vi "BMU诊断标定.vi"(8 "CAN端口":u16(ring), 9 "设备索引号":u16(ring), 10 "CAN卡类型":u32(ring)=21) -> ()   [LabVIEW 2013] (continued)
                n1433 = Build Array(w1898, w1897, w1896, w1895, w1894, w1893) -> (w1899:bool[])
                n1434 = Build Array(w1907, w1906, w1905, w1904, w1903, w1902) -> (w1901:bool[])
                n1435 = And Array Elements(Boolean array=w1899) -> (logical AND=w1892:bool)
                n1436 = And Array Elements(Boolean array=w1901) -> (logical AND=w1900:bool)
                n1437 = Not(x=w1891) -> (.not. x?=w1915:bool)
              }
              frame "电池包信息1" {
                w1920 = 2
                w1928 = 2
                w1919 = 2
                w1917 = FALSE ("1 6")
                n1438 = Select(t=0, s=w1925, f=1) -> (s? t:f=w1918:i32)
                n1439 = property on="串联数" class="DigNum (严格)"("Disabled"=w1918) -> ()  [unwired: 2 in, 2 out]
                n1440 = property on="并联数" class="DigNum (严格)"("Disabled"=w1918) -> ()  [unwired: 2 in, 2 out]
                n1441 = property on="电池厂家" class="DigNum (严格)"("Disabled"=w1918) -> ()  [unwired: 2 in, 2 out]
                n1442 = property on="电池类型" class="DigNum (严格)"("Disabled"=w1918) -> ()  [unwired: 2 in, 2 out]
                n1443 = property on="额定能量" class="DigNum (严格)"("Disabled"=w1918) -> ()  [unwired: 2 in, 2 out]
                n1444 = property on="额定容量" class="DigNum (严格)"("Disabled"=w1918) -> ()  [unwired: 2 in, 2 out]
                n1445 = property on="实际容量" class="DigNum (严格)"("Disabled"=w1918) -> ()  [unwired: 2 in, 2 out]
                n1446 = property on="电池组信息" class="Clust (严格)"("Disabled"=w1918) -> ()  [unwired: 2 in, 2 out]
                n1447 = property on="生产日期" class="Str"("DisabledEnum"=w1918) -> ()  [unwired: 2 in, 2 out]
                n1448 = property on="车牌号" class="Str"("DisabledEnum"=w1919) -> ()  [unwired: 2 in, 2 out]
                n1449 = property on="产权标识" class="DigNum (严格)"("Disabled"=w1918) -> ()  [unwired: 2 in, 2 out]
                n1450 = property on="应用车型" class="DigNum (严格)"("Disabled"=w1918) -> ()  [unwired: 2 in, 2 out]
                n1451 = property on="额定总压" class="DigNum (严格)"("Disabled"=w1918) -> ()  [unwired: 2 in, 2 out]
                n1452 = property on="电池包序号" class="DigNum (严格)"("DisabledEnum"=w1918) -> ()  [unwired: 2 in, 2 out]
                n1453 = property on="电池包组号" class="DigNum (严格)"("DisabledEnum"=w1919) -> ()  [unwired: 2 in, 2 out]
                n1454 = property on="最大允许单体电压" class="DigNum (严格)"("Disabled"=w1928) -> ()  [unwired: 2 in, 2 out]
                n1455 = property on="最大允许总电压" class="DigNum (严格)"("Disabled"=w1928) -> ()  [unwired: 2 in, 2 out]
                n1456 = property on="最大允许温度" class="DigNum (严格)"("Disabled"=w1928) -> ()  [unwired: 2 in, 2 out]
                n1457 = property on="最小允许温度" class="DigNum (严格)"("Disabled"=w1928) -> ()  [unwired: 2 in, 2 out]
                n1458 = property on="最大允许充电电流" class="DigNum (严格)"("Disabled"=w1928) -> ()  [unwired: 2 in, 2 out]
                n1459 = property on="最小允许充电电流" class="DigNum (严格)"("Disabled"=w1928) -> ()  [unwired: 2 in, 2 out]
                n1460 = property on="最小允许单体电压" class="DigNum (严格)"("Disabled"=w1928) -> ()  [unwired: 2 in, 2 out]
                n1461 = property on="电流步长" class="DigNum (严格)"("Disabled"=w1928) -> ()  [unwired: 2 in, 2 out]
                n1462 = property on="SOC" class="DigNum (严格)"("Disabled"=w1928) -> ()  [unwired: 2 in, 2 out]
                n1463 = property on="充电总安时" class="DigNum (严格)"("Disabled"=w1928) -> ()  [unwired: 2 in, 2 out]
                n1464 = property on="放电总安时" class="DigNum (严格)"("Disabled"=w1928) -> ()  [unwired: 2 in, 2 out]
                n1465 = property on="放空次数" class="DigNum (严格)"("DisabledEnum"=w1920) -> ()  [unwired: 2 in, 2 out]
                n1466 = property on="充满次数" class="DigNum (严格)"("DisabledEnum"=w1920) -> ()  [unwired: 2 in, 2 out]
                n1467 = property on="充电次数" class="DigNum (严格)"("DisabledEnum"=w1920) -> ()  [unwired: 2 in, 2 out]
                n1468 = global read "功能码全局.vi" "24"() -> (w1923:bool[])
                n1469 = global read "功能码全局.vi" "23"() -> (w1924:bool[])
                n1470 = Index Array(array=w1923) -> (element #3=w1921:bool)  [unwired: 8 in, 7 out]
                n1471 = Index Array(array=w1924) -> (element #3=w1922:bool)  [unwired: 8 in, 7 out]
                n1472 = Not(x=w1917) -> (.not. x?=w1929:bool)
              }
              frame "电池包组号" {
                w1934 = 2
                w1933 = 2
                w1943 = 2
                w1935 = 2
                w1944 = 2
                w1931 = FALSE ("1 6")
                n1473 = property on="串联数" class="DigNum (严格)"("Disabled"=w1944) -> ()  [unwired: 2 in, 2 out]
                n1474 = property on="并联数" class="DigNum (严格)"("Disabled"=w1944) -> ()  [unwired: 2 in, 2 out]
                n1475 = property on="电池厂家" class="DigNum (严格)"("Disabled"=w1944) -> ()  [unwired: 2 in, 2 out]
                n1476 = property on="电池类型" class="DigNum (严格)"("Disabled"=w1944) -> ()  [unwired: 2 in, 2 out]
                n1477 = property on="额定能量" class="DigNum (严格)"("Disabled"=w1944) -> ()  [unwired: 2 in, 2 out]
                n1478 = property on="额定容量" class="DigNum (严格)"("Disabled"=w1944) -> ()  [unwired: 2 in, 2 out]
                n1479 = property on="实际容量" class="DigNum (严格)"("Disabled"=w1944) -> ()  [unwired: 2 in, 2 out]
                n1480 = Select(t=0, s=w1940, f=1) -> (s? t:f=w1932:i32)
                n1481 = property on="生产日期" class="Str"("DisabledEnum"=w1934) -> ()  [unwired: 2 in, 2 out]
                n1482 = property on="电池包序号" class="DigNum (严格)"("DisabledEnum"=w1934) -> ()  [unwired: 2 in, 2 out]
                n1483 = property on="车牌号" class="Str"("DisabledEnum"=w1934) -> ()  [unwired: 2 in, 2 out]
                n1484 = property on="电池包组号" class="DigNum (严格)"("DisabledEnum"=w1932) -> ()  [unwired: 2 in, 2 out]
                n1485 = property on="电池组信息" class="Clust (严格)"("Disabled"=w1932) -> ()  [unwired: 2 in, 2 out]
                n1486 = property on="产权标识" class="DigNum (严格)"("Disabled"=w1935) -> ()  [unwired: 2 in, 2 out]
                n1487 = property on="应用车型" class="DigNum (严格)"("Disabled"=w1935) -> ()  [unwired: 2 in, 2 out]
                n1488 = property on="额定总压" class="DigNum (严格)"("Disabled"=w1935) -> ()  [unwired: 2 in, 2 out]
                n1489 = property on="放空次数" class="DigNum (严格)"("DisabledEnum"=w1933) -> ()  [unwired: 2 in, 2 out]
                n1490 = property on="充满次数" class="DigNum (严格)"("DisabledEnum"=w1933) -> ()  [unwired: 2 in, 2 out]
                n1491 = property on="充电次数" class="DigNum (严格)"("DisabledEnum"=w1933) -> ()  [unwired: 2 in, 2 out]
                n1492 = property on="最大允许单体电压" class="DigNum (严格)"("Disabled"=w1943) -> ()  [unwired: 2 in, 2 out]
                n1493 = property on="最大允许总电压" class="DigNum (严格)"("Disabled"=w1943) -> ()  [unwired: 2 in, 2 out]
                n1494 = property on="最大允许温度" class="DigNum (严格)"("Disabled"=w1943) -> ()  [unwired: 2 in, 2 out]
                n1495 = property on="最小允许温度" class="DigNum (严格)"("Disabled"=w1943) -> ()  [unwired: 2 in, 2 out]
                n1496 = property on="最大允许充电电流" class="DigNum (严格)"("Disabled"=w1943) -> ()  [unwired: 2 in, 2 out]
                n1497 = property on="最小允许充电电流" class="DigNum (严格)"("Disabled"=w1943) -> ()  [unwired: 2 in, 2 out]
                n1498 = property on="最小允许单体电压" class="DigNum (严格)"("Disabled"=w1943) -> ()  [unwired: 2 in, 2 out]
                n1499 = property on="电流步长" class="DigNum (严格)"("Disabled"=w1943) -> ()  [unwired: 2 in, 2 out]
                n1500 = property on="SOC" class="DigNum (严格)"("Disabled"=w1943) -> ()  [unwired: 2 in, 2 out]
                n1501 = property on="充电总安时" class="DigNum (严格)"("Disabled"=w1943) -> ()  [unwired: 2 in, 2 out]
                n1502 = property on="放电总安时" class="DigNum (严格)"("Disabled"=w1943) -> ()  [unwired: 2 in, 2 out]
                n1503 = global read "功能码全局.vi" "24"() -> (w1938:bool[])
                n1504 = global read "功能码全局.vi" "23"() -> (w1939:bool[])
                n1505 = Index Array(array=w1938) -> (element #3=w1936:bool)  [unwired: 8 in, 7 out]
                n1506 = Index Array(array=w1939) -> (element #3=w1937:bool)  [unwired: 8 in, 7 out]
                n1507 = Not(x=w1931) -> (.not. x?=w1945:bool)
              }
              frame "充放电安时" {
                w1949 = 2
                w1948 = 2
                w1958 = 2
                w1959 = 2
                w1961 = 2
                w1947 = FALSE ("1 6")
                n1508 = property on="串联数" class="DigNum (严格)"("Disabled"=w1961) -> ()  [unwired: 2 in, 2 out]
                n1509 = property on="并联数" class="DigNum (严格)"("Disabled"=w1961) -> ()  [unwired: 2 in, 2 out]
                n1510 = property on="电池厂家" class="DigNum (严格)"("Disabled"=w1961) -> ()  [unwired: 2 in, 2 out]
                n1511 = property on="电池类型" class="DigNum (严格)"("Disabled"=w1961) -> ()  [unwired: 2 in, 2 out]
                n1512 = property on="额定能量" class="DigNum (严格)"("Disabled"=w1961) -> ()  [unwired: 2 in, 2 out]
                n1513 = property on="额定容量" class="DigNum (严格)"("Disabled"=w1961) -> ()  [unwired: 2 in, 2 out]
                n1514 = property on="实际容量" class="DigNum (严格)"("Disabled"=w1961) -> ()  [unwired: 2 in, 2 out]
                n1515 = Select(t=0, s=w1955, f=1) -> (s? t:f=w1954:i32)
                n1516 = property on="生产日期" class="Str"("DisabledEnum"=w1949) -> ()  [unwired: 2 in, 2 out]
                n1517 = property on="电池包序号" class="DigNum (严格)"("DisabledEnum"=w1949) -> ()  [unwired: 2 in, 2 out]
                n1518 = property on="车牌号" class="Str"("DisabledEnum"=w1949) -> ()  [unwired: 2 in, 2 out]
                n1519 = property on="电池包组号" class="DigNum (严格)"("DisabledEnum"=w1949) -> ()  [unwired: 2 in, 2 out]
                n1520 = property on="电池组信息" class="Clust (严格)"("Disabled"=w1954) -> ()  [unwired: 2 in, 2 out]
                n1521 = property on="额定总压" class="DigNum (严格)"("Disabled"=2) -> ()  [unwired: 2 in, 2 out]
                n1522 = property on="产权标识" class="DigNum (严格)"("Disabled"=w1959) -> ()  [unwired: 2 in, 2 out]
                n1523 = property on="应用车型" class="DigNum (严格)"("Disabled"=w1959) -> ()  [unwired: 2 in, 2 out]
                n1524 = property on="放空次数" class="DigNum (严格)"("DisabledEnum"=w1948) -> ()  [unwired: 2 in, 2 out]
                n1525 = property on="充满次数" class="DigNum (严格)"("DisabledEnum"=w1948) -> ()  [unwired: 2 in, 2 out]
                n1526 = property on="充电次数" class="DigNum (严格)"("DisabledEnum"=w1948) -> ()  [unwired: 2 in, 2 out]
                n1527 = property on="最大允许单体电压" class="DigNum (严格)"("Disabled"=w1958) -> ()  [unwired: 2 in, 2 out]
                n1528 = property on="最大允许总电压" class="DigNum (严格)"("Disabled"=w1958) -> ()  [unwired: 2 in, 2 out]
                n1529 = property on="最大允许温度" class="DigNum (严格)"("Disabled"=w1958) -> ()  [unwired: 2 in, 2 out]
                n1530 = property on="最小允许温度" class="DigNum (严格)"("Disabled"=w1958) -> ()  [unwired: 2 in, 2 out]
                n1531 = property on="最大允许充电电流" class="DigNum (严格)"("Disabled"=w1958) -> ()  [unwired: 2 in, 2 out]
                n1532 = property on="最小允许充电电流" class="DigNum (严格)"("Disabled"=w1958) -> ()  [unwired: 2 in, 2 out]
                n1533 = property on="最小允许单体电压" class="DigNum (严格)"("Disabled"=w1958) -> ()  [unwired: 2 in, 2 out]
                n1534 = property on="电流步长" class="DigNum (严格)"("Disabled"=w1958) -> ()  [unwired: 2 in, 2 out]
                n1535 = property on="SOC" class="DigNum (严格)"("Disabled"=w1958) -> ()  [unwired: 2 in, 2 out]
                n1536 = property on="充电总安时" class="DigNum (严格)"("Disabled"=w1954) -> ()  [unwired: 2 in, 2 out]
                n1537 = property on="放电总安时" class="DigNum (严格)"("Disabled"=w1954) -> ()  [unwired: 2 in, 2 out]
                n1538 = Not(x=w1947) -> (.not. x?=w1962:bool)
                n1539 = global read "功能码全局.vi" "24"() -> (w1952:bool[])
                n1540 = global read "功能码全局.vi" "23"() -> (w1953:bool[])
                n1541 = Index Array(array=w1952) -> (element #7=w1950:bool)  [unwired: 8 in, 7 out]
                n1542 = Index Array(array=w1953) -> (element #7=w1951:bool)  [unwired: 8 in, 7 out]
              }
              frame "充电次数" {
                w1967 = 2
                w1976 = 2
                w1977 = 2
                w1968 = 2
                w1978 = 2
                w1964 = FALSE ("1 6")
                n1543 = property on="串联数" class="DigNum (严格)"("Disabled"=w1978) -> ()  [unwired: 2 in, 2 out]
                n1544 = property on="并联数" class="DigNum (严格)"("Disabled"=w1978) -> ()  [unwired: 2 in, 2 out]
                n1545 = property on="电池厂家" class="DigNum (严格)"("Disabled"=w1978) -> ()  [unwired: 2 in, 2 out]
                n1546 = property on="电池类型" class="DigNum (严格)"("Disabled"=w1978) -> ()  [unwired: 2 in, 2 out]
                n1547 = property on="额定能量" class="DigNum (严格)"("Disabled"=w1978) -> ()  [unwired: 2 in, 2 out]
                n1548 = property on="额定容量" class="DigNum (严格)"("Disabled"=w1978) -> ()  [unwired: 2 in, 2 out]
                n1549 = property on="实际容量" class="DigNum (严格)"("Disabled"=w1978) -> ()  [unwired: 2 in, 2 out]
                n1550 = Select(t=0, s=w1973, f=1) -> (s? t:f=w1965:i32)
                n1551 = property on="生产日期" class="Str"("DisabledEnum"=w1967) -> ()  [unwired: 2 in, 2 out]
                n1552 = property on="电池包序号" class="DigNum (严格)"("DisabledEnum"=w1967) -> ()  [unwired: 2 in, 2 out]
                n1553 = property on="车牌号" class="Str"("DisabledEnum"=w1967) -> ()  [unwired: 2 in, 2 out]
                n1554 = property on="电池组信息" class="Clust (严格)"("Disabled"=w1965) -> ()  [unwired: 2 in, 2 out]
                n1555 = property on="电池包组号" class="DigNum (严格)"("DisabledEnum"=w1967) -> ()  [unwired: 2 in, 2 out]
                n1556 = property on="额定总压" class="DigNum (严格)"("Disabled"=w1968) -> ()  [unwired: 2 in, 2 out]
                n1557 = property on="产权标识" class="DigNum (严格)"("Disabled"=w1968) -> ()  [unwired: 2 in, 2 out]
                n1558 = property on="应用车型" class="DigNum (严格)"("Disabled"=w1968) -> ()  [unwired: 2 in, 2 out]
                n1559 = property on="放空次数" class="DigNum (严格)"("DisabledEnum"=w1965) -> (error out=w1966:errorcluster)  [unwired: 2 in, 1 out]
                n1560 = property on="充满次数" class="DigNum (严格)"("DisabledEnum"=w1965) -> ()  [unwired: 2 in, 2 out]
                n1561 = property on="充电次数" class="DigNum (严格)"("DisabledEnum"=w1965) -> ()  [unwired: 2 in, 2 out]
                n1562 = property on="最大允许单体电压" class="DigNum (严格)"("Disabled"=w1977) -> ()  [unwired: 2 in, 2 out]
                n1563 = property on="最大允许总电压" class="DigNum (严格)"("Disabled"=w1977) -> ()  [unwired: 2 in, 2 out]
                n1564 = property on="最大允许温度" class="DigNum (严格)"("Disabled"=w1977) -> ()  [unwired: 2 in, 2 out]
                n1565 = property on="最小允许温度" class="DigNum (严格)"("Disabled"=w1977) -> ()  [unwired: 2 in, 2 out]
                n1566 = property on="最大允许充电电流" class="DigNum (严格)"("Disabled"=w1977) -> ()  [unwired: 2 in, 2 out]
                n1567 = property on="最小允许充电电流" class="DigNum (严格)"(error in=w1966, "Disabled"=w1977) -> ()  [unwired: 1 in, 2 out]
                n1568 = property on="最小允许单体电压" class="DigNum (严格)"("Disabled"=w1977) -> ()  [unwired: 2 in, 2 out]
                n1569 = property on="电流步长" class="DigNum (严格)"("Disabled"=w1977) -> ()  [unwired: 2 in, 2 out]
                n1570 = property on="SOC" class="DigNum (严格)"("Disabled"=w1977) -> ()  [unwired: 2 in, 2 out]
                n1571 = property on="充电总安时" class="DigNum (严格)"("Disabled"=w1976) -> ()  [unwired: 2 in, 2 out]
                n1572 = property on="放电总安时" class="DigNum (严格)"("Disabled"=w1976) -> ()  [unwired: 2 in, 2 out]
                n1573 = Not(x=w1964) -> (.not. x?=w1979:bool)
                n1574 = global read "功能码全局.vi" "24"() -> (w1971:bool[])
                n1575 = global read "功能码全局.vi" "23"() -> (w1972:bool[])
                n1576 = Index Array(array=w1971) -> (element #8=w1970:bool)  [unwired: 8 in, 7 out]
                n1577 = Index Array(array=w1972) -> (element #8=w1969:bool)  [unwired: 8 in, 7 out]
              }
              frame "SOC" {
                w1983 = 2
                w1982 = 2
                w1992 = 2
                w1993 = 2
                w1994 = 2
                w1996 = 2
                w1981 = FALSE ("1 6")
                n1578 = property on="串联数" class="DigNum (严格)"("Disabled"=w1996) -> ()  [unwired: 2 in, 2 out]
                n1579 = property on="并联数" class="DigNum (严格)"("Disabled"=w1996) -> ()  [unwired: 2 in, 2 out]
                n1580 = property on="电池厂家" class="DigNum (严格)"("Disabled"=w1996) -> ()  [unwired: 2 in, 2 out]
                n1581 = property on="电池类型" class="DigNum (严格)"("Disabled"=w1996) -> ()  [unwired: 2 in, 2 out]
                n1582 = property on="额定能量" class="DigNum (严格)"("Disabled"=w1996) -> ()  [unwired: 2 in, 2 out]
                n1583 = property on="额定容量" class="DigNum (严格)"("Disabled"=w1996) -> ()  [unwired: 2 in, 2 out]
                n1584 = property on="实际容量" class="DigNum (严格)"("Disabled"=w1996) -> ()  [unwired: 2 in, 2 out]
                n1585 = Select(t=0, s=w1989, f=1) -> (s? t:f=w1988:i32)
                n1586 = property on="生产日期" class="Str"("DisabledEnum"=w1983) -> ()  [unwired: 2 in, 2 out]
                n1587 = property on="电池包序号" class="DigNum (严格)"("DisabledEnum"=w1983) -> ()  [unwired: 2 in, 2 out]
                n1588 = property on="车牌号" class="Str"("DisabledEnum"=w1983) -> ()  [unwired: 2 in, 2 out]
                n1589 = property on="电池包组号" class="DigNum (严格)"("DisabledEnum"=w1983) -> ()  [unwired: 2 in, 2 out]
                n1590 = property on="电池组信息" class="Clust (严格)"("Disabled"=w1988) -> ()  [unwired: 2 in, 2 out]
                n1591 = property on="SOC" class="DigNum (严格)"("Disabled"=w1988) -> ()  [unwired: 2 in, 2 out]
                n1592 = property on="额定总压" class="DigNum (严格)"("Disabled"=2) -> ()  [unwired: 2 in, 2 out]
                n1593 = property on="产权标识" class="DigNum (严格)"("Disabled"=w1994) -> ()  [unwired: 2 in, 2 out]
                n1594 = property on="应用车型" class="DigNum (严格)"("Disabled"=w1994) -> ()  [unwired: 2 in, 2 out]
                n1595 = property on="放空次数" class="DigNum (严格)"("DisabledEnum"=w1982) -> ()  [unwired: 2 in, 2 out]
                n1596 = property on="充满次数" class="DigNum (严格)"("DisabledEnum"=w1982) -> ()  [unwired: 2 in, 2 out]
                n1597 = property on="充电次数" class="DigNum (严格)"("DisabledEnum"=w1982) -> ()  [unwired: 2 in, 2 out]
                n1598 = property on="最大允许单体电压" class="DigNum (严格)"("Disabled"=w1993) -> ()  [unwired: 2 in, 2 out]
                n1599 = property on="最大允许总电压" class="DigNum (严格)"("Disabled"=w1993) -> ()  [unwired: 2 in, 2 out]
                n1600 = property on="最大允许温度" class="DigNum (严格)"("Disabled"=w1993) -> ()  [unwired: 2 in, 2 out]
                n1601 = property on="最小允许温度" class="DigNum (严格)"("Disabled"=w1993) -> ()  [unwired: 2 in, 2 out]
                n1602 = property on="最大允许充电电流" class="DigNum (严格)"("Disabled"=w1993) -> ()  [unwired: 2 in, 2 out]
                n1603 = property on="最小允许充电电流" class="DigNum (严格)"("Disabled"=w1993) -> ()  [unwired: 2 in, 2 out]
                n1604 = property on="最小允许单体电压" class="DigNum (严格)"("Disabled"=w1993) -> ()  [unwired: 2 in, 2 out]
                n1605 = property on="电流步长" class="DigNum (严格)"("Disabled"=w1993) -> ()  [unwired: 2 in, 2 out]
                n1606 = property on="充电总安时" class="DigNum (严格)"("Disabled"=w1992) -> ()  [unwired: 2 in, 2 out]
                n1607 = property on="放电总安时" class="DigNum (严格)"("Disabled"=w1992) -> ()  [unwired: 2 in, 2 out]
                n1608 = Not(x=w1981) -> (.not. x?=w1997:bool)
                n1609 = global read "功能码全局.vi" "24"() -> (w1986:bool[])
                n1610 = global read "功能码全局.vi" "23"() -> (w1987:bool[])
                n1611 = Index Array(array=w1986) -> (element #6=w1985:bool)  [unwired: 8 in, 7 out]
                n1612 = Index Array(array=w1987) -> (element #6=w1984:bool)  [unwired: 8 in, 7 out]
              }
              frame "车牌号" {
                w2002 = 2
                w2001 = 2
                w2011 = 2
                w2012 = 2
                w2013 = 2
                w2015 = 2
                w1999 = FALSE ("1 6")
                n1613 = property on="串联数" class="DigNum (严格)"("Disabled"=w2015) -> ()  [unwired: 2 in, 2 out]
                n1614 = property on="并联数" class="DigNum (严格)"("Disabled"=w2015) -> ()  [unwired: 2 in, 2 out]
                n1615 = property on="电池厂家" class="DigNum (严格)"("Disabled"=w2015) -> ()  [unwired: 2 in, 2 out]
                n1616 = property on="电池类型" class="DigNum (严格)"("Disabled"=w2015) -> ()  [unwired: 2 in, 2 out]
                n1617 = property on="额定能量" class="DigNum (严格)"("Disabled"=w2015) -> ()  [unwired: 2 in, 2 out]
                n1618 = property on="额定容量" class="DigNum (严格)"("Disabled"=w2015) -> ()  [unwired: 2 in, 2 out]
                n1619 = property on="实际容量" class="DigNum (严格)"("Disabled"=w2015) -> ()  [unwired: 2 in, 2 out]
                n1620 = Select(t=0, s=w2007, f=1) -> (s? t:f=w2000:i32)
                n1621 = property on="生产日期" class="Str"("DisabledEnum"=w2002) -> ()  [unwired: 2 in, 2 out]
                n1622 = property on="电池包序号" class="DigNum (严格)"("DisabledEnum"=w2002) -> ()  [unwired: 2 in, 2 out]
                n1623 = property on="电池包组号" class="DigNum (严格)"("DisabledEnum"=w2002) -> ()  [unwired: 2 in, 2 out]
                n1624 = property on="电池组信息" class="Clust (严格)"("Disabled"=w2000) -> ()  [unwired: 2 in, 2 out]
                n1625 = property on="车牌号" class="Str"("DisabledEnum"=w2000) -> ()  [unwired: 2 in, 2 out]
                n1626 = property on="额定总压" class="DigNum (严格)"("Disabled"=2) -> ()  [unwired: 2 in, 2 out]
                n1627 = property on="产权标识" class="DigNum (严格)"("Disabled"=w2013) -> ()  [unwired: 2 in, 2 out]
                n1628 = property on="应用车型" class="DigNum (严格)"("Disabled"=w2013) -> ()  [unwired: 2 in, 2 out]
                n1629 = property on="放空次数" class="DigNum (严格)"("DisabledEnum"=w2001) -> ()  [unwired: 2 in, 2 out]
                n1630 = property on="充满次数" class="DigNum (严格)"("DisabledEnum"=w2001) -> ()  [unwired: 2 in, 2 out]
                n1631 = property on="充电次数" class="DigNum (严格)"("DisabledEnum"=w2001) -> ()  [unwired: 2 in, 2 out]
                n1632 = property on="最大允许单体电压" class="DigNum (严格)"("Disabled"=w2012) -> ()  [unwired: 2 in, 2 out]
                n1633 = property on="最大允许总电压" class="DigNum (严格)"("Disabled"=w2012) -> ()  [unwired: 2 in, 2 out]
                n1634 = property on="最大允许温度" class="DigNum (严格)"("Disabled"=w2012) -> ()  [unwired: 2 in, 2 out]
                n1635 = property on="最小允许温度" class="DigNum (严格)"("Disabled"=w2012) -> ()  [unwired: 2 in, 2 out]
                n1636 = property on="最大允许充电电流" class="DigNum (严格)"("Disabled"=w2012) -> ()  [unwired: 2 in, 2 out]
                n1637 = property on="最小允许充电电流" class="DigNum (严格)"("Disabled"=w2012) -> ()  [unwired: 2 in, 2 out]
                n1638 = property on="最小允许单体电压" class="DigNum (严格)"("Disabled"=w2012) -> ()  [unwired: 2 in, 2 out]
                n1639 = property on="电流步长" class="DigNum (严格)"("Disabled"=w2012) -> ()  [unwired: 2 in, 2 out]
                n1640 = property on="SOC" class="DigNum (严格)"("Disabled"=2) -> ()  [unwired: 2 in, 2 out]
                n1641 = property on="充电总安时" class="DigNum (严格)"("Disabled"=w2011) -> ()  [unwired: 2 in, 2 out]
                n1642 = property on="放电总安时" class="DigNum (严格)"("Disabled"=w2011) -> ()  [unwired: 2 in, 2 out]
                n1643 = Not(x=w1999) -> (.not. x?=w2016:bool)
                n1644 = global read "功能码全局.vi" "24"() -> (w2005:bool[])
                n1645 = global read "功能码全局.vi" "23"() -> (w2006:bool[])
                n1646 = Index Array(array=w2005) -> (element #5=w2003:bool)  [unwired: 8 in, 7 out]
                n1647 = Index Array(array=w2006) -> (element #5=w2004:bool)  [unwired: 8 in, 7 out]
              }
              frame "充电参数" {
                w2020 = 2
                w2019 = 2
                w2029 = 2
                w2030 = 2
                w2032 = 2
                w2018 = FALSE ("1 6")
                n1648 = property on="串联数" class="DigNum (严格)"("Disabled"=w2032) -> ()  [unwired: 2 in, 2 out]
                n1649 = property on="并联数" class="DigNum (严格)"("Disabled"=w2032) -> ()  [unwired: 2 in, 2 out]
                n1650 = property on="电池厂家" class="DigNum (严格)"("Disabled"=w2032) -> ()  [unwired: 2 in, 2 out]
                n1651 = property on="电池类型" class="DigNum (严格)"("Disabled"=w2032) -> ()  [unwired: 2 in, 2 out]
                n1652 = property on="额定能量" class="DigNum (严格)"("Disabled"=w2032) -> ()  [unwired: 2 in, 2 out]
                n1653 = property on="额定容量" class="DigNum (严格)"("Disabled"=w2032) -> ()  [unwired: 2 in, 2 out]
                n1654 = property on="实际容量" class="DigNum (严格)"("Disabled"=w2032) -> ()  [unwired: 2 in, 2 out]
                n1655 = Select(t=0, s=w2026, f=1) -> (s? t:f=w2025:i32)
                n1656 = property on="生产日期" class="Str"("DisabledEnum"=w2020) -> ()  [unwired: 2 in, 2 out]
                n1657 = property on="电池包序号" class="DigNum (严格)"("DisabledEnum"=w2020) -> ()  [unwired: 2 in, 2 out]
                n1658 = property on="车牌号" class="Str"("DisabledEnum"=w2020) -> ()  [unwired: 2 in, 2 out]
                n1659 = property on="电池组信息" class="Clust (严格)"("Disabled"=w2025) -> ()  [unwired: 2 in, 2 out]
                n1660 = property on="电池包组号" class="DigNum (严格)"("DisabledEnum"=w2020) -> ()  [unwired: 2 in, 2 out]
                n1661 = property on="额定总压" class="DigNum (严格)"("Disabled"=2) -> ()  [unwired: 2 in, 2 out]
                n1662 = property on="产权标识" class="DigNum (严格)"("Disabled"=w2030) -> ()  [unwired: 2 in, 2 out]
                n1663 = property on="应用车型" class="DigNum (严格)"("Disabled"=w2030) -> ()  [unwired: 2 in, 2 out]
                n1664 = property on="放空次数" class="DigNum (严格)"("DisabledEnum"=w2019) -> ()  [unwired: 2 in, 2 out]
                n1665 = property on="充满次数" class="DigNum (严格)"("DisabledEnum"=w2019) -> ()  [unwired: 2 in, 2 out]
                n1666 = property on="充电次数" class="DigNum (严格)"("DisabledEnum"=w2019) -> ()  [unwired: 2 in, 2 out]
                n1667 = property on="最大允许单体电压" class="DigNum (严格)"("Disabled"=w2025) -> ()  [unwired: 2 in, 2 out]
                n1668 = property on="最大允许总电压" class="DigNum (严格)"("Disabled"=w2025) -> ()  [unwired: 2 in, 2 out]
                n1669 = property on="最大允许温度" class="DigNum (严格)"("Disabled"=w2025) -> ()  [unwired: 2 in, 2 out]
                n1670 = property on="最小允许温度" class="DigNum (严格)"("Disabled"=w2025) -> ()  [unwired: 2 in, 2 out]
                n1671 = property on="最大允许充电电流" class="DigNum (严格)"("Disabled"=w2025) -> ()  [unwired: 2 in, 2 out]
                n1672 = property on="最小允许充电电流" class="DigNum (严格)"("Disabled"=w2025) -> ()  [unwired: 2 in, 2 out]
                n1673 = property on="最小允许单体电压" class="DigNum (严格)"("Disabled"=w2025) -> ()  [unwired: 2 in, 2 out]
                n1674 = property on="电流步长" class="DigNum (严格)"("Disabled"=w2025) -> ()  [unwired: 2 in, 2 out]
                n1675 = property on="SOC" class="DigNum (严格)"("Disabled"=w2029) -> ()  [unwired: 2 in, 2 out]
                n1676 = property on="充电总安时" class="DigNum (严格)"("Disabled"=w2029) -> ()  [unwired: 2 in, 2 out]
                n1677 = property on="放电总安时" class="DigNum (严格)"("Disabled"=w2029) -> ()  [unwired: 2 in, 2 out]
                n1678 = Not(x=w2018) -> (.not. x?=w2033:bool)
                n1679 = global read "功能码全局.vi" "24"() -> (w2023:bool[])
                n1680 = global read "功能码全局.vi" "23"() -> (w2024:bool[])
                n1681 = Index Array(array=w2023) -> (element #4=w2021:bool)  [unwired: 8 in, 7 out]
                n1682 = Index Array(array=w2024) -> (element #4=w2022:bool)  [unwired: 8 in, 7 out]
              }
              frame "均衡参数" {
                w2035 = FALSE ("1 6")
                n1683 = Select(t=0, s=w2041, f=1) -> (s? t:f=w2039:i32)
                n1684 = property on="均衡计算-电压高阀值1级" class="DigNum (严格)"("DisabledEnum"=w2039) -> ()  [unwired: 2 in, 2 out]
                n1685 = property on="均衡计算-电压高阀值2级" class="DigNum (严格)"("DisabledEnum"=w2039) -> ()  [unwired: 2 in, 2 out]
                n1686 = property on="均衡计算-电压低阀值1级" class="DigNum (严格)"("DisabledEnum"=w2039) -> ()  [unwired: 2 in, 2 out]
                n1687 = property on="均衡计算-电压低阀值2级" class="DigNum (严格)"("DisabledEnum"=w2039) -> ()  [unwired: 2 in, 2 out]
                n1688 = property on="均衡计算-最低电压阀值" class="DigNum (严格)"("DisabledEnum"=w2039) -> ()  [unwired: 2 in, 2 out]
                n1689 = property on="均衡停止-最低电压阀值" class="DigNum (严格)"("DisabledEnum"=w2039) -> ()  [unwired: 2 in, 2 out]
                n1690 = property on="均衡计算-电压极差阀值" class="DigNum (严格)"("DisabledEnum"=w2039) -> ()  [unwired: 2 in, 2 out]
                n1691 = property on="均衡参数" class="Clust (严格)"("DisabledEnum"=w2039) -> ()  [unwired: 2 in, 2 out]
                n1692 = property on="充电结束电压(90%)" class="DigNum (严格)"("DisabledEnum"=w2039) -> ()  [unwired: 2 in, 2 out]
                n1693 = property on="充电结束电压(91%)" class="DigNum (严格)"("DisabledEnum"=w2039) -> ()  [unwired: 2 in, 2 out]
                n1694 = property on="充电结束电压(92%)" class="DigNum (严格)"("DisabledEnum"=w2039) -> ()  [unwired: 2 in, 2 out]
                n1695 = property on="充电结束电压(93%)" class="DigNum (严格)"("DisabledEnum"=w2039) -> ()  [unwired: 2 in, 2 out]
                n1696 = property on="充电结束电压(94%)" class="DigNum (严格)"("DisabledEnum"=w2039) -> ()  [unwired: 2 in, 2 out]
                n1697 = property on="充电结束电压(95%)" class="DigNum (严格)"("DisabledEnum"=w2039) -> ()  [unwired: 2 in, 2 out]
                n1698 = property on="充电结束电压(96%)" class="DigNum (严格)"("DisabledEnum"=w2039) -> ()  [unwired: 2 in, 2 out]
                n1699 = property on="充电结束电压(97%)" class="DigNum (严格)"("DisabledEnum"=w2039) -> ()  [unwired: 2 in, 2 out]
                n1700 = property on="充电结束电压(98%)" class="DigNum (严格)"("DisabledEnum"=w2039) -> ()  [unwired: 2 in, 2 out]
                n1701 = property on="充电结束电压(99%)" class="DigNum (严格)"("DisabledEnum"=w2039) -> ()  [unwired: 2 in, 2 out]
                n1702 = property on="充电结束电压(100%)" class="DigNum (严格)"("DisabledEnum"=w2039) -> ()  [unwired: 2 in, 2 out]
                n1703 = disable-structure shown="启用" {
                  disable-tunnel: [w2045 w2047] -> w2038
                  disable-tunnel: [w2044 w2047] -> w2037
                  frame Enabled {
                    n1704 = global read "功能码全局.vi" "18"() -> (w2046:bool[])
                    n1705 = Index Array(array=w2046) -> (element #1=w2045:bool, element #2=w2044:bool)  [unwired: 8 in, 6 out]
                  }
                  frame Disabled {
                    w2047 = TRUE
                  }
                }
                n1706 = Not(x=w2035) -> (.not. x?=w2036:bool)
              }
              frame "均衡阀值" {
                w2050 = 2
                w2048 = FALSE ("1 6")
                n1707 = Select(t=0, s=w2055, f=1) -> (s? t:f=w2053:i32)
                n1708 = property on="均衡计算-电压高阀值1级" class="DigNum (严格)"("DisabledEnum"=w2053) -> ()  [unwired: 2 in, 2 out]
                n1709 = property on="均衡计算-电压高阀值2级" class="DigNum (严格)"("DisabledEnum"=w2053) -> ()  [unwired: 2 in, 2 out]
                n1710 = property on="均衡计算-电压低阀值1级" class="DigNum (严格)"("DisabledEnum"=w2053) -> ()  [unwired: 2 in, 2 out]
                n1711 = property on="均衡计算-电压低阀值2级" class="DigNum (严格)"("DisabledEnum"=w2053) -> ()  [unwired: 2 in, 2 out]
                n1712 = property on="均衡计算-最低电压阀值" class="DigNum (严格)"("DisabledEnum"=w2053) -> ()  [unwired: 2 in, 2 out]
                n1713 = property on="均衡停止-最低电压阀值" class="DigNum (严格)"("DisabledEnum"=w2053) -> ()  [unwired: 2 in, 2 out]
                n1714 = property on="均衡计算-电压极差阀值" class="DigNum (严格)"("DisabledEnum"=w2053) -> ()  [unwired: 2 in, 2 out]
                n1715 = property on="均衡参数" class="Clust (严格)"("DisabledEnum"=w2053) -> ()  [unwired: 2 in, 2 out]
                n1716 = property on="充电结束电压(90%)" class="DigNum (严格)"("DisabledEnum"=w2050) -> ()  [unwired: 2 in, 2 out]
                n1717 = property on="充电结束电压(91%)" class="DigNum (严格)"("DisabledEnum"=w2050) -> ()  [unwired: 2 in, 2 out]
                n1718 = property on="充电结束电压(92%)" class="DigNum (严格)"("DisabledEnum"=w2050) -> ()  [unwired: 2 in, 2 out]
                n1719 = property on="充电结束电压(93%)" class="DigNum (严格)"("DisabledEnum"=w2050) -> ()  [unwired: 2 in, 2 out]
                n1720 = property on="充电结束电压(94%)" class="DigNum (严格)"("DisabledEnum"=w2050) -> ()  [unwired: 2 in, 2 out]
                n1721 = property on="充电结束电压(95%)" class="DigNum (严格)"("DisabledEnum"=w2050) -> ()  [unwired: 2 in, 2 out]
                n1722 = property on="充电结束电压(96%)" class="DigNum (严格)"("DisabledEnum"=w2050) -> ()  [unwired: 2 in, 2 out]
                n1723 = property on="充电结束电压(97%)" class="DigNum (严格)"("DisabledEnum"=w2050) -> ()  [unwired: 2 in, 2 out]
                n1724 = property on="充电结束电压(98%)" class="DigNum (严格)"("DisabledEnum"=w2050) -> ()  [unwired: 2 in, 2 out]
                n1725 = property on="充电结束电压(99%)" class="DigNum (严格)"("DisabledEnum"=w2050) -> ()  [unwired: 2 in, 2 out]
                n1726 = property on="充电结束电压(100%)" class="DigNum (严格)"("DisabledEnum"=w2050) -> ()  [unwired: 2 in, 2 out]
                n1727 = disable-structure shown="启用" {
                  disable-tunnel: [w2059 w2061] -> w2052
                  disable-tunnel: [w2058 w2061] -> w2051
                  frame Enabled {
                    n1728 = global read "功能码全局.vi" "18"() -> (w2060:bool[])
                    n1729 = Index Array(array=w2060) -> (element #1=w2059:bool, element #2=w2058:bool)  [unwired: 8 in, 6 out]
                  }
                  frame Disabled {
                    w2061 = TRUE
                  }
                }
                n1730 = Not(x=w2048) -> (.not. x?=w2049:bool)
              }
              frame "充电结束电压" {
                w2065 = 2
                w2062 = FALSE ("1 6")
                n1731 = Select(t=0, s=w2069, f=1) -> (s? t:f=w2064:i32)
                n1732 = property on="均衡计算-电压高阀值1级" class="DigNum (严格)"("DisabledEnum"=w2065) -> ()  [unwired: 2 in, 2 out]
                n1733 = property on="均衡计算-电压高阀值2级" class="DigNum (严格)"("DisabledEnum"=w2065) -> ()  [unwired: 2 in, 2 out]
                n1734 = property on="均衡计算-电压低阀值1级" class="DigNum (严格)"("DisabledEnum"=w2065) -> ()  [unwired: 2 in, 2 out]
                n1735 = property on="均衡计算-电压低阀值2级" class="DigNum (严格)"("DisabledEnum"=w2065) -> ()  [unwired: 2 in, 2 out]
                n1736 = property on="均衡计算-最低电压阀值" class="DigNum (严格)"("DisabledEnum"=w2065) -> ()  [unwired: 2 in, 2 out]
                n1737 = property on="均衡停止-最低电压阀值" class="DigNum (严格)"("DisabledEnum"=w2065) -> ()  [unwired: 2 in, 2 out]
                n1738 = property on="均衡计算-电压极差阀值" class="DigNum (严格)"("DisabledEnum"=w2065) -> ()  [unwired: 2 in, 2 out]
                n1739 = property on="均衡参数" class="Clust (严格)"("DisabledEnum"=w2064) -> ()  [unwired: 2 in, 2 out]
                n1740 = property on="充电结束电压(90%)" class="DigNum (严格)"("DisabledEnum"=w2064) -> ()  [unwired: 2 in, 2 out]
                n1741 = property on="充电结束电压(91%)" class="DigNum (严格)"("DisabledEnum"=w2064) -> ()  [unwired: 2 in, 2 out]
                n1742 = property on="充电结束电压(92%)" class="DigNum (严格)"("DisabledEnum"=w2064) -> ()  [unwired: 2 in, 2 out]
                n1743 = property on="充电结束电压(93%)" class="DigNum (严格)"("DisabledEnum"=w2064) -> ()  [unwired: 2 in, 2 out]
                n1744 = property on="充电结束电压(94%)" class="DigNum (严格)"("DisabledEnum"=w2064) -> ()  [unwired: 2 in, 2 out]
                n1745 = property on="充电结束电压(95%)" class="DigNum (严格)"("DisabledEnum"=w2064) -> ()  [unwired: 2 in, 2 out]
                n1746 = property on="充电结束电压(96%)" class="DigNum (严格)"("DisabledEnum"=w2064) -> ()  [unwired: 2 in, 2 out]
                n1747 = property on="充电结束电压(97%)" class="DigNum (严格)"("DisabledEnum"=w2064) -> ()  [unwired: 2 in, 2 out]
                n1748 = property on="充电结束电压(98%)" class="DigNum (严格)"("DisabledEnum"=w2064) -> ()  [unwired: 2 in, 2 out]
                n1749 = property on="充电结束电压(99%)" class="DigNum (严格)"("DisabledEnum"=w2064) -> ()  [unwired: 2 in, 2 out]
                n1750 = property on="充电结束电压(100%)" class="DigNum (严格)"("DisabledEnum"=w2064) -> ()  [unwired: 2 in, 2 out]
                n1751 = disable-structure shown="启用" {
                  disable-tunnel: [w2073 w2075] -> w2067
                  disable-tunnel: [w2072 w2075] -> w2066
                  frame Enabled {
                    n1752 = global read "功能码全局.vi" "18"() -> (w2074:bool[])
                    n1753 = Index Array(array=w2074) -> (element #1=w2073:bool, element #2=w2072:bool)  [unwired: 8 in, 6 out]
                  }
                  frame Disabled {
                    w2075 = TRUE
                  }
                }
                n1754 = Not(x=w2062) -> (.not. x?=w2063:bool)
              }
              frame "假", Default {
                w2076 = FALSE ("1 6")
                n1755 = Not(x=w2076) -> (.not. x?=w2077:bool)
              }
            }
            n1756 = local write "等级 2"(w1667) -> ()
            n1757 = local write "1 6"(w1666) -> ()
            n1758 = local write "1 7"(w1665) -> ()
            n1759 = local write "1 8"(w1664) -> ()
            n1760 = local write "1 9"(w1663) -> ()
            n1761 = local write "1 10"(w1662) -> ()
            n1762 = local write "1 12"(w1656) -> ()
            n1763 = property on="单个读取" class="Bool (严格)"("Visible"=w1661) -> ()  [unwired: 2 in, 2 out]
            n1764 = property on="单个写入" class="Bool (严格)"("Visible"=w1660) -> ()  [unwired: 2 in, 2 out]
          }
          event "从板个数": Value Change {
            n1765 = event-data() -> ()  [unwired: 7 out]
            n1766 = local read "从板个数"() -> (w2079:dbl)
            n1767 = call "多从板对应参数-new.vi"("从板个数"=w2079) -> ("输出数组"=w2080:string[])  [unwired: 1 in]
            n1768 = control-ref of="项目信息"() -> (w2081:refnum<vi>)
            n1769 = stacked-sequence {
              tunnel: w2081 -> [_ w2088 w2092]
              tunnel: w2080 -> [_ w2087 w2091]
              frame #0 {
                n1770 = local write "项目信息"(string[][] [] ("项目信息")) -> ()
              }
              frame #1 {
                n1771 = call "表格数据输入-8.6.vi"("行数"=u32 0, "列数"=u32 0, "字符串数组"=w2087, "表格引用"=w2088) -> ()  [unwired: 8 out]
              }
              frame #2 {
                n1772 = Array Size(array=w2091) -> (size(s)=w2090:i32)
                n1773 = for {
                  N: w2090 -> [_]
                  tunnel: [""] -> w2089 mode=indexing
                }
                n1774 = call "表格数据输入-8.6.vi"("行数"=u32 0, "列数"=u32 1, "字符串数组"=w2089, "表格引用"=w2092) -> ()  [unwired: 8 out]
              }
            }
          }
          event "主界面选项": Value Change {
            n1775 = event-data() -> ("NewVal"=w2096:enum32{"单选选项1", "单选选项2", "单选选项2 2", "单选选项2 3"})  [unwired: 6 out]
            n1776 = control-ref of="单选选项2 2"() -> (w2101:refnum<vi>)
            n1777 = control-ref of="单选选项2"() -> (w2103:refnum<vi>)
            n1778 = control-ref of="单选选项1"() -> (w2102:refnum<vi>)
            n1779 = control-ref of="单选选项2 3"() -> (w2097:refnum<vi>)
            n1780 = Build Array(w2102, w2103, w2101, w2097) -> (w2100:refnum<vi>[])
            n1781 = case shown="\"单选选项2 3\"" w2096 {
              selector: w2096 -> [w2114 w2119 w2124 w2129]
              tunnel: w2100 -> [w2115 w2120 w2125 w2130]
              tunnel: [w2113 w2118 w2123 w2128] -> w2106
              tunnel: [w2112 w2117 w2122 w2127] -> w2105
              tunnel: [enum32{"读写参数", "版本读取", "其它诊断"}."读写参数" ("选项卡控件 2") enum32{"读写参数", "版本读取", "其它诊断"}."版本读取" ("选项卡控件 2") enum32{"读写参数", "版本读取", "其它诊断"}."其它诊断" ("选项卡控件 2") enum32{"读写参数", "版本读取", "其它诊断", "高压板校正"}."高压板校正" ("选项卡控件 2")] -> w2104
              frame "单选选项1", Default {
                n1782 = Delete From Array(array=w2115, index=w2114) -> (deleted portion=w2112:refnum<vi>, array with subset deleted=w2113:refnum<vi>[])  [unwired: 1 in]
              }
              frame "单选选项2" {
                n1783 = Delete From Array(array=w2120, index=w2119) -> (deleted portion=w2117:refnum<vi>, array with subset deleted=w2118:refnum<vi>[])  [unwired: 1 in]
              }
              frame "单选选项2 2" {
                n1784 = Delete From Array(array=w2125, index=w2124) -> (deleted portion=w2122:refnum<vi>, array with subset deleted=w2123:refnum<vi>[])  [unwired: 1 in]
              }
              frame "单选选项2 3" {
                n1785 = Delete From Array(array=w2130, index=w2129) -> (deleted portion=w2127:refnum<vi>, array with subset deleted=w2128:refnum<vi>[])  [unwired: 1 in]
              }
            }
            n1786 = local write "面板选择"(w2104) -> ()
            n1787 = for {
              tunnel: u32 16777215 -> [w2110]
              tunnel: w2106 -> [w2109] mode=indexing
              n1788 = property class="Bool (严格)"(reference=w2109, "BoolText.TextColor"=w2110) -> ()  [unwired: 1 in, 2 out]
            }
            n1789 = property class="Bool (严格)"(reference=w2105, "BoolText.TextColor"=u32 65511) -> ()  [unwired: 1 in, 2 out]
          }
          event "主从板": Value Change {
            w2132 = FALSE ("可见")
            n1790 = event-data() -> ()  [unwired: 7 out]
            n1791 = control-ref of="单选选项2"() -> (w2140:refnum<vi>)
            n1792 = control-ref of="单选选项1"() -> (w2139:refnum<vi>)
            n1793 = local read "主从板"() -> (w2147:enum32{"单选选项2", "单选选项1"})
            n1794 = Build Array(w2140, w2139) -> (w2146:refnum<vi>[])
            n1795 = case shown="\"单选选项2\"" w2147 {
              selector: w2147 -> [w2192 w2235]
              tunnel: w2146 -> [w2193 w2234]
              tunnel: [enum32{"主板", "从板"}."主板" ("主从选择") enum32{"主板", "从板"}."从板" ("主从选择")] -> w2145
              tunnel: [w2191 w2233] -> w2142
              tunnel: [w2190 w2232] -> w2141
              tunnel: [TRUE FALSE] -> w2137
              tunnel: [w2151 w2212] -> w2134
              tunnel: [w2152 w2217] -> w2133
              tunnel: [FALSE ("可见") TRUE ("可见")] -> w2131
              frame "单选选项1", Default {
                n1796 = global read "功能码全局.vi" "主板项目信息7"() -> (w2163:bool[])
                n1797 = global read "功能码全局.vi" "主板项目信息4"() -> (w2186:bool[])
                n1798 = global read "功能码全局.vi" "主板控制类信息10"() -> (w2167:bool[])
                n1799 = global read "功能码全局.vi" "主板故障阀值9"() -> (w2164:bool[])
                n1800 = global read "功能码全局.vi" "主板项目信息5"() -> (w2177:bool[])
                n1801 = global read "功能码全局.vi" "主板项目信息6"() -> (w2187:bool[])
                n1802 = global read "功能码全局.vi" "主板版本号11"() -> (w2178:bool[])
                n1803 = Delete From Array(array=w2187, length=1 ("长度"), index=0 ("索引")) -> (deleted portion=w2176:bool[], array with subset deleted=w2159:bool[])
                n1804 = Index Array(array=w2186, index #1=5 ("索引"), index #2=6 ("索引")) -> (element #1=w2175:bool, element #2=w2158:bool)
                n1805 = Index Array(array=w2178) -> (element #1=w2171:bool, element #2=w2154:bool)  [unwired: 2 in]
                n1806 = Array Subset(array=w2164, index=2 ("索引"), length=3 ("长度")) -> (w2173:bool[])
                n1807 = Delete From Array(array=w2163, length=3 ("索引"), index=2 ("长度")) -> (deleted portion=w2174:bool[], array with subset deleted=w2157:bool[])
                n1808 = Array Subset(array=w2167, index=4 ("索引"), length=2 ("长度")) -> (w2172:bool[])
                n1809 = Delete From Array(array=w2193, index=w2192) -> (deleted portion=w2190:refnum<vi>, array with subset deleted=w2191:refnum<vi>[])  [unwired: 1 in]
                n1810 = Insert Into Array(array=w2177, new element #1=w2176, new element #2=w2175, new element #3=w2174, new element #4=w2173, new element #5=w2172, new element #6=w2171) -> (w2170:bool[])  [unwired: 1 in]
                n1811 = Array Subset(array=w2167, index=6 ("索引"), length=2 ("长度")) -> (w2155:bool[])
                n1812 = Array Subset(array=w2164, index=5 ("索引"), length=3 ("长度")) -> (w2156:bool[])
                n1813 = And Array Elements(Boolean array=w2170) -> (logical AND=w2152:bool)
                n1814 = Insert Into Array(array=w2159, new element #1=w2158, new element #2=w2157, new element #3=w2156, new element #4=w2155, new element #5=w2154) -> (w2153:bool[])  [unwired: 1 in]
                n1815 = And Array Elements(Boolean array=w2153) -> (logical AND=w2151:bool)
              }
              frame "单选选项2" {
                n1816 = global read "功能码全局.vi" "18"() -> (w2208:bool[])
                n1817 = global read "功能码全局.vi" "15"() -> (w2229:bool[])
                n1818 = global read "功能码全局.vi" "16"() -> (w2226:bool[])
                n1819 = Delete From Array(array=w2234, index=w2235) -> (deleted portion=w2232:refnum<vi>, array with subset deleted=w2233:refnum<vi>[])  [unwired: 1 in]
                n1820 = Index Array(array=w2226, index #1=4 ("索引"), index #2=5 ("索引"), index #3=6 ("索引"), index #4=7 ("索引")) -> (element #1=w2220:bool, element #2=w2219:bool, element #3=w2215:bool, element #4=w2214:bool)
                n1821 = Index Array(array=w2208, index #1=4 ("索引"), index #2=5 ("索引"), index #3=6 ("索引"), index #4=7 ("索引"), index #5=2 ("索引"), index #6=3 ("索引"), index #7=0 ("索引"), index #8=1 ("索引")) -> (element #1=w2201:bool, element #2=w2204:bool, element #3=w2203:bool, element #4=w2202:bool, element #5=w2200:bool, element #6=w2199:bool, element #7=w2194:bool, element #8=w2195:bool)
                n1822 = Delete From Array(array=w2229, length=4 ("长度"), index=0 ("索引")) -> (deleted portion=w2221:bool[], array with subset deleted=w2216:bool[])
                n1823 = Insert Into Array(array=w2216, new element #1=w2215, new element #2=w2214, new element #3=w2204, new element #4=w2203, new element #5=w2202, new element #6=w2195) -> (w2213:bool[])  [unwired: 1 in]
                n1824 = Insert Into Array(array=w2221, new element #1=w2220, new element #2=w2219, new element #3=w2201, new element #4=w2200, new element #5=w2199, new element #6=w2194) -> (w2218:bool[])  [unwired: 1 in]
                n1825 = And Array Elements(Boolean array=w2218) -> (logical AND=w2217:bool)
                n1826 = And Array Elements(Boolean array=w2213) -> (logical AND=w2212:bool)
              }
            }
            n1827 = property on="全部写入" class="Bool (严格)"("Visible"=w2134) -> ()  [unwired: 2 in, 2 out]
            n1828 = property on="全部读取" class="Bool (严格)"("Visible"=w2133) -> ()  [unwired: 2 in, 2 out]
            n1829 = property on="从板号" class="DigNum (严格)"("Visible"=w2131) -> ()  [unwired: 2 in, 2 out]
            n1830 = local write "主从选择"(w2145) -> ()
            n1831 = property on="从板个数" class="DigNum (严格)"("Visible"=w2137) -> ()  [unwired: 2 in, 2 out]
            n1832 = for {
              tunnel: u32 87470 -> [w2149]
              tunnel: w2142 -> [w2148] mode=indexing
              n1833 = property class="Bool (严格)"(reference=w2148, "BoolText.TextColor"=w2149) -> ()  [unwired: 1 in, 2 out]
            }
            n1834 = Not(x=w2137) -> (.not. x?=w2138:bool)
            n1835 = property class="Bool (严格)"(reference=w2141, "BoolText.TextColor"=u32 16777215) -> ()  [unwired: 1 in, 2 out]
            n1836 = property on="主板选项" class="Tree (严格)"("Visible"=w2137) -> ()  [unwired: 2 in, 2 out]
            n1837 = property on="从板选项" class="Tree (严格)"("Visible"=w2138) -> ()  [unwired: 2 in, 2 out]
            n1838 = property on="当前从板板号" class="DigNum (严格)"("Visible"=w2138) -> ()  [unwired: 2 in, 2 out]
            n1839 = property on="单个读取" class="Bool (严格)"("Visible"=w2132) -> ()  [unwired: 2 in, 2 out]
            n1840 = property on="单个写入" class="Bool (严格)"("Visible"=w2132) -> ()  [unwired: 2 in, 2 out]
          }
          event "从板号": Value Change {
            n1841 = event-data() -> ()  [unwired: 7 out]
            n1842 = local read "key names"() -> (w2237:string[])
            n1843 = Empty Array?(array=w2237) -> (empty?=w2236:bool)
            n1844 = case shown="假" w2236 {
              tunnel: w2237 -> [w2240 _]
              frame False {
                n1845 = stacked-sequence {
                  seq-local: [w2241 _] -> [_ w2304]
                  tunnel: w2240 -> [w2249 _]
                  frame #0 {
                    w2280 = 2 ("长度")
                    w2277 = 20 ("长度")
                    w2265 = 1 ("索引")
                    n1846 = local read "从板号"() -> (w2241:u8)
                    n1847 = local read "输出数组"() -> (w2250:string[][])
                    n1848 = Decrement(x=w2241) -> (x-1=w2247:u8)
                    n1849 = Index Array(array=w2250, index (col)=w2247) -> (element=w2278:string[])  [unwired: 1 in]
                    n1850 = global write "读配置文件全局2.vi" "从板板号"(w2241) -> ()
                    n1851 = Search 1D Array(1D array=w2249, element="风机开启温度" ("元素")) -> (index of element=w2262:i32)  [unwired: 1 in]
                    n1852 = Search 1D Array(1D array=w2249, element="电压过高一级" ("元素"), start index (0)=w2262) -> (index of element=w2260:i32)
                    n1853 = Decrement(x=w2262) -> (x-1=w2264:i32)
                    n1854 = Array Subset(array=w2278, index=w2265, length=w2264) -> (w2248:string[])
                    n1855 = Array Subset(array=w2278, index=w2260, length=21 ("长度")) -> (w2252:string[])
                    n1856 = Array Subset(array=w2249, index=w2265, length=w2264) -> (w2295:string[])
                    n1857 = Array Subset(array=w2278, index=w2262, length=7 ("长度")) -> (w2258:string[])
                    n1858 = for {
                      tunnel: w2252 -> [w2297] mode=indexing
                      tunnel: [w2296] -> w2251 mode=indexing
                      n1859 = Fract/Exp String To Number(string=w2297) -> (number=w2296:dbl)  [unwired: 3 in, 1 out]
                    }
                    n1860 = for {
                      tunnel: w2258 -> [w2299] mode=indexing
                      tunnel: [w2298] -> w2242 mode=indexing
                      n1861 = Fract/Exp String To Number(string=w2299) -> (number=w2298:dbl)  [unwired: 3 in, 1 out]
                    }
                    n1862 = Delete From Array(array=w2251, length=7 ("长度"), index=0 ("索引")) -> (deleted portion=w2245:dbl[], array with subset deleted=w2255:dbl[])
                    n1863 = Array To Cluster(array=w2242) -> (cluster=w2267:T20)
                    n1864 = global write "读配置文件全局2.vi" "加热控制参数"(w2242) -> ()
                    n1865 = Delete From Array(array=w2255, length=7 ("长度"), index=0 ("索引")) -> (deleted portion=w2244:dbl[], array with subset deleted=w2243:dbl[])
                    n1866 = local write "加热控制参数"(w2267) -> ()
                    n1867 = Array To Cluster(array=w2245) -> (cluster=w2292:T20)
                    n1868 = Array To Cluster(array=w2243) -> (cluster=w2294:T20)
                    n1869 = Array To Cluster(array=w2244) -> (cluster=w2293:T20)
                    n1870 = global write "读配置文件全局2.vi" "三级故障阀值"(w2243) -> ()
                    n1871 = global write "读配置文件全局2.vi" "一级故障阀值"(w2245) -> ()
                    n1872 = global write "读配置文件全局2.vi" "二级故障阀值"(w2244) -> ()
                    n1873 = local write "一级故障 6"(w2292) -> ()
                    n1874 = local write "一级故障 8"(w2294) -> ()
                    n1875 = local write "一级故障 7"(w2293) -> ()
                    n1876 = Search 1D Array(1D array=w2295, element="温度个数" ("元素")) -> (index of element=w2274:i32)  [unwired: 1 in]
                    n1877 = Search 1D Array(1D array=w2295, element="第一个保险通道" ("元素")) -> (index of element=w2275:i32)  [unwired: 1 in]
                    n1878 = Search 1D Array(1D array=w2295, element="电压个数" ("元素")) -> (index of element=w2273:i32)  [unwired: 1 in]
                    n1879 = Search 1D Array(1D array=w2295, element="第1通道电压个数" ("元素")) -> (index of element=w2276:i32)  [unwired: 1 in]
                    n1880 = Array Subset(array=w2248, index=w2273, length=2 ("长度")) -> (w2281:string[])
                    n1881 = Array Subset(array=w2248, index=w2274, length=w2280) -> (w2283:string[])
                    n1882 = Array Subset(array=w2248, index=w2275, length=20 ("长度")) -> (w2284:string[])
                    n1883 = Array Subset(array=w2248, index=w2276, length=w2277) -> (w2282:string[])
                    n1884 = Insert Into Array(array=w2281, new element #1=w2282, new element #2=w2283, new element #3=w2284) -> (w2246:string[])  [unwired: 1 in]
                    n1885 = Array Subset(array=w2295, index=w2273, length=w2280) -> (w2285:string[])
                    n1886 = Array Subset(array=w2295, index=w2274, length=w2280) -> (w2287:string[])
                    n1887 = Array Subset(array=w2295, index=w2275, length=w2277) -> (w2288:string[])
                    n1888 = Array Subset(array=w2295, index=w2276, length=w2277) -> (w2286:string[])
                    n1889 = global write "读配置文件全局2.vi" "表格"(w2246) -> ()
                    n1890 = Insert Into Array(array=w2285, new element #1=w2286, new element #2=w2287, new element #3=w2288) -> (w2290:string[])  [unwired: 1 in]
                    n1891 = Build Array(w2290, w2246) -> (w2289:string[][])
                    n1892 = Transpose 2D Array(2D array=w2289) -> (transposed array=w2291:string[][])
                    n1893 = local write "项目信息 2"(w2291) -> ()
                  }
                  frame #1 {
                    n1894 = Number To Decimal String(number=w2304) -> (decimal integer string=w2302:string)  [unwired: 1 in]
                    n1895 = control-ref of="结果"() -> (w2307:refnum<vi>)
                    n1896 = Concatenate Strings("从板", w2302, "导入完成") -> (w2300:string)
                    n1897 = Build Array(w2300) -> (w2305:string[])
                    n1898 = call "表格编辑.vi"("新元素/子数组"=w2305, "活动单元格:单元格背景色"=u32 6618880, "MCListbox引用句柄"=w2307) -> ()  [unwired: 9 out]
                  }
                }
              }
              frame True {
              }
            }
          }
          event "读配置文件": Value Change {
            n1899 = event-data() -> ("NewVal"=w2308:bool)  [unwired: 6 out]
            n1900 = case shown="真" w2308 {
              tunnel: w2312 -> [w2314 w2320]
              tunnel: [w2314 w2319] -> w2311
              tunnel: w2310 -> [w2313 w2318]
              tunnel: [w2313 w2317] -> w2309
              frame False {
              }
              frame True {
                n1901 = local write "布尔"(TRUE ("布尔")) -> ()
                n1902 = Enqueue Element(queue=w2320, element="读配置文件", error in (no error)=w2318) -> (queue out=w2319:refnum<queue>, error out=w2317:errorcluster)  [unwired: 2 out]
              }
            }
          }
